vi "Check LabVIEW RT Installed.vi"(8 "error in":errorcluster) -> (0 "error out":errorcluster, 1 "registry labview path":path, 2 "registry subkey used":string, 3 "labview version":string, 4 "rt folder path":path, 6 "labview rt installed?":bool)   [LabVIEW 2026]
doc: "Reads the current LabVIEW version from an Application Property Node, builds the versioned registry key, reads install path, and checks whether TargetsIT exists."
uses:
  <vilib>/registry/registry.llb/Registry SAM.ctl
  <vilib>/registry/registry.llb/Read Registry Value Simple STR.vi
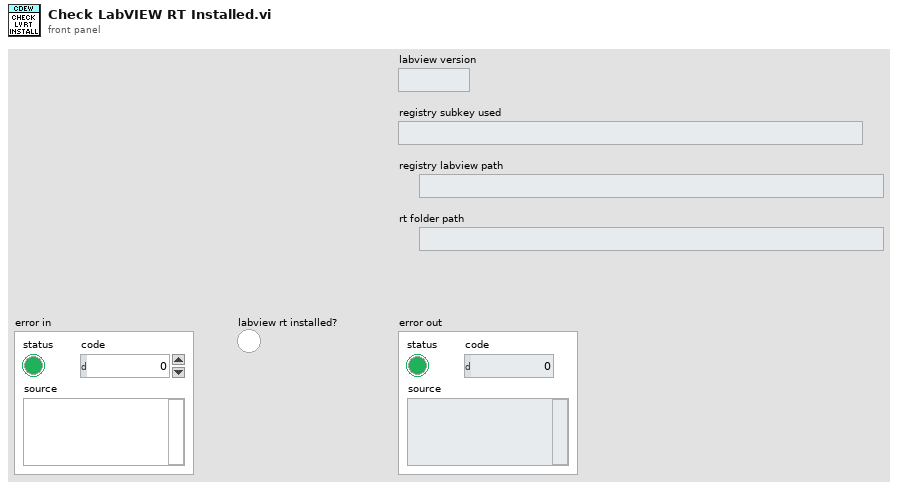
[diagram p1: front panel]
types:
  T1 = typedef "Registry SAM.ctl" = enum32{"KEY_QUERY_VALUE", "KEY_SET_VALUE", "KEY_CREATE_SUB_KEY", "KEY_ENUMERATE_SUB_KEYS", "KEY_NOTIFY", "KEY_CREATE_LINK", "KEY_READ", "KEY_WRITE", "KEY_ALL_ACCESS", "KEY_READ | KEY_WRITE"}
  T2 = typedef "Registry refnum.ctl" = refnum<k1>
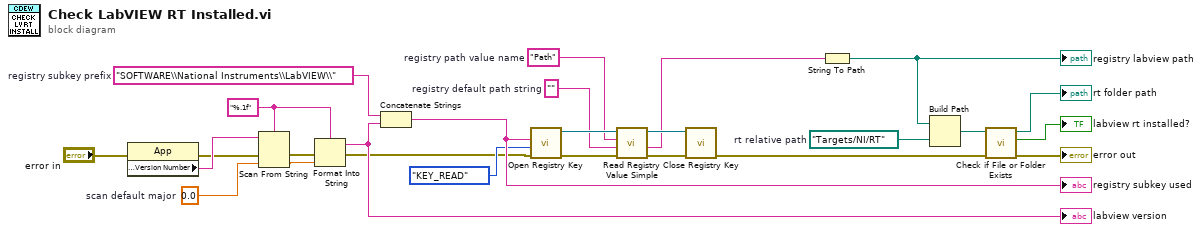
[diagram p0: block diagram]
diagram:
  w5 = "%.1f" ("format string")
  w8 = 0.0  # scan default major
  w15 = path "Targets/NI/RT"  # rt relative path
  w21 = ""  # registry default path string
  w22 = "Path"  # registry path value name
  w25 = "SOFTWARE\\National Instruments\\LabVIEW\\"  # registry subkey prefix
  n1 = property class="App"(error in="error in") -> (error out=w3:errorcluster, "Application:Version Number"=w7:string)  [unwired: 1 in, 1 out]
  n2 = Scan From String(format string=w5, input string=w7, error in=w3, default 1=w8) -> (error out=w2:errorcluster, output 1=w6:dbl)  [unwired: 1 in, 2 out]
  n3 = Format Into String(format string=w5, error in=w2, w6) -> (resulting string=w4:string, error out=w1:errorcluster)  [unwired: 1 in]
  "labview version" <- w4
  n4 = Concatenate Strings(w25, w4) -> (w24:string)
  "registry subkey used" <- w24
  n5 = call <vilib>:"Open Registry Key.vi"("error in (no error)"=w1, "security access mask (KEY_READ | KEY_WRITE)"=Registry_SAM."KEY_READ", "subkey"=w24) -> ("error out"=w20:errorcluster, "refnum out"=w23:T2)  [unwired: 7 in]
  n6 = call-poly <vilib>:"Read Registry Value Simple.vi"("error in (no error)"=w20, "default data"=w21, "value"=w22, "refnum"=w23) -> ("error out"=w18:errorcluster, "String/Binary data"=w17:string, "refnum out"=w19:T2)  [unwired: 2 in, 1 out]
  n7 = call <vilib>:"Close Registry Key.vi"("error in (no error)"=w18, "refnum"=w19) -> ("error out"=w13:errorcluster)  [unwired: 5 in]
  n8 = String To Path(string=w17) -> (path=w16:path)
  "registry labview path" <- w16
  n9 = Build Path(base path=w16, name or relative path=w15) -> (appended path=w14:path)
  n10 = call <vilib>:"Check if File or Folder Exists.vi"("error in (no error)"=w13, "path"=w14) -> ("error out"=→"error out":errorcluster, "file or folder exists?"=→"labview rt installed?":bool, "dup path"=→"rt folder path":path)  [unwired: 7 in]
